vi "Update DropdownMenu.vi"(10 "VacuumLines Obj":refnum<class "VacuumLines.lvclass">, 11 "Ref of Array":refnum<vi>) -> ()   [LabVIEW 2016, in "Hardware.lvlib" / "VacuumLine.lvlib" / "VacuumLines Configuration.lvclass"]
uses:
  <userlib>/Common Components/Hardware/Abstract System/VacuumLine/VacuumLines Configuration/VacuumLines Configuration.lvclass
  <userlib>/Common Components/Hardware/Abstract System/VacuumLine/VacuumLines/VacuumLines.lvclass
  <userlib>/Common Components/Hardware/Abstract System/VacuumLine/VacuumLines/VacuumLines.lvclass/VacuumLines.ctl
  <userlib>/Common Components/Hardware/Abstract Hardware/Hardware.lvclass/Hardware.ctl
  <userlib>/Common Components/Hardware/Abstract System/VacuumLine/VacuumLine/VacuumLine.lvclass/VacuumLine.ctl
  <userlib>/Common Components/Hardware/GaugeController/GaugeController/GaugeController.lvclass
  C:/Program Files (x86)/National Instruments/LabVIEW 2016/user.lib/Common Components/Hardware/Abstract Hardware/Hardware.lvclass
  <userlib>/Common Components/Hardware/Abstract System/VacuumLine/VacuumLine/VacuumLine.lvclass
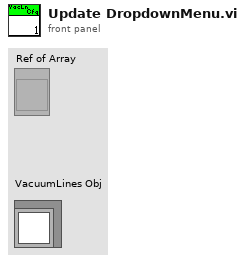
[diagram p1: front panel]
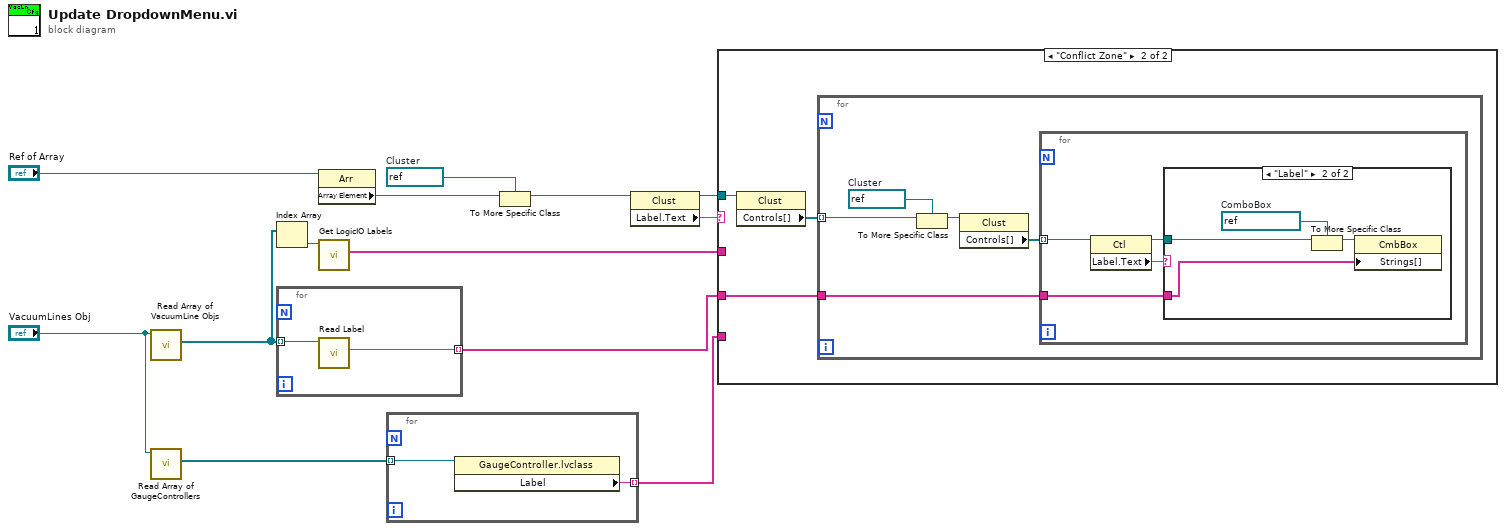
[diagram p0: block diagram]
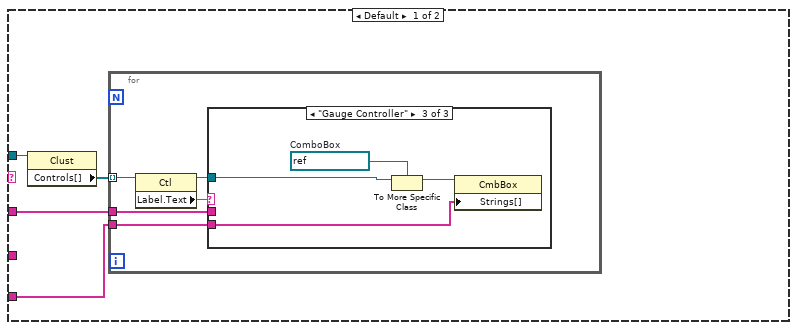
[diagram p2: hidden frame]
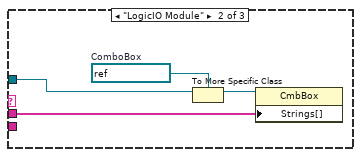
[diagram p4: hidden frame]
diagram:
  w12 = refnum<vi> refnum  # Cluster
  n1 = call <userlib>:"Read Array of VacuumLine Objs.vi"("VacuumLines in"="VacuumLines Obj") -> ("Array of VacuumLine Objs"=w4:refnum<class "VacuumLine.lvclass">[])  [unwired: 9 in, 1 out]
  n2 = call <userlib>:"Read Array of GaugeControllers.vi"("VacuumLines in"="VacuumLines Obj") -> ("Array of GaugeControllers"=w7:refnum<class "GaugeController.lvclass">[])  [unwired: 9 in, 1 out]
  n3 = Index Array(array=w4) -> (element=w8:refnum<class "VacuumLine.lvclass">)  [unwired: 1 in]
  n4 = for {
    tunnel: w4 -> [w15] mode=indexing
    tunnel: [w14] -> w3 mode=indexing
    n5 = call <userlib>:"Read Label.vi"("VacuumLine in"=w15) -> ("Label"=w14:string)  [unwired: 8 in, 2 out]
  }
  n6 = property class="Arr"(reference="Ref of Array") -> ("Array Element"=w11:refnum<vi>)  [unwired: 1 in, 2 out]
  n7 = call <userlib>:"Get LogicIO Labels.vi"("VacuumLine in"=w8) -> ("LogicIO Labels"=w13:string[])  [unwired: 8 in, 2 out]
  n8 = for {
    tunnel: w7 -> [w17] mode=indexing
    tunnel: [w16] -> w6 mode=indexing
    n9 = property class="GaugeController.lvclass"(reference=w17) -> ("Label"=w16:string)  [unwired: 1 in, 2 out]
  }
  n10 = To More Specific Class(target class=w12, reference=w11) -> (specific class reference=w10:refnum<vi>)  [unwired: 1 in, 1 out]
  n11 = property class="Clust"(reference=w10) -> (reference out=w2:refnum<vi>, "Label.Text"=w1:string)  [unwired: 1 in, 1 out]
  n12 = case shown="\"Conflict Zone\"" w1 {
    tunnel: w13 -> [w21 _]
    tunnel: w6 -> [w19 _]
    tunnel: w3 -> [_ w35]
    tunnel: w2 -> [w18 w36]
    frame Default {
      n13 = property class="Clust"(reference=w18) -> ("Controls[]"=w20:refnum<vi>[])  [unwired: 1 in, 2 out]
      n14 = for {
        tunnel: w20 -> [w26] mode=indexing
        tunnel: w21 -> [w23]
        tunnel: w19 -> [w22]
        n15 = property class="Ctl"(reference=w26) -> (reference out=w24:refnum<vi>, "Label.Text"=w25:string)  [unwired: 1 in, 1 out]
        n16 = case shown="\"Gauge Controller\"" w25 {
          tunnel: w24 -> [_ w28 w32]
          tunnel: w23 -> [_ w27 _]
          tunnel: w22 -> [_ _ w31]
          frame Default {
          }
          frame "LogicIO Module" {
            w30 = refnum<vi> refnum  # ComboBox
            n17 = To More Specific Class(target class=w30, reference=w28) -> (specific class reference=w29:refnum<vi>)  [unwired: 1 in, 1 out]
            n18 = property class="CmbBox"(reference=w29, "Strings[]"=w27) -> ()  [unwired: 1 in, 2 out]
          }
          frame "Gauge Controller" {
            w34 = refnum<vi> refnum  # ComboBox
            n19 = To More Specific Class(target class=w34, reference=w32) -> (specific class reference=w33:refnum<vi>)  [unwired: 1 in, 1 out]
            n20 = property class="CmbBox"(reference=w33, "Strings[]"=w31) -> ()  [unwired: 1 in, 2 out]
          }
        }
      }
    }
    frame "Conflict Zone" {
      n21 = property class="Clust"(reference=w36) -> ("Controls[]"=w37:refnum<vi>[])  [unwired: 1 in, 2 out]
      n22 = for {
        tunnel: w37 -> [w39] mode=indexing
        tunnel: w35 -> [w42]
        w41 = refnum<vi> refnum  # Cluster
        n23 = To More Specific Class(target class=w41, reference=w39) -> (specific class reference=w40:refnum<vi>)  [unwired: 1 in, 1 out]
        n24 = property class="Clust"(reference=w40) -> ("Controls[]"=w38:refnum<vi>[])  [unwired: 1 in, 2 out]
        n25 = for {
          tunnel: w42 -> [w44]
          tunnel: w38 -> [w43] mode=indexing
          n26 = property class="Ctl"(reference=w43) -> (reference out=w45:refnum<vi>, "Label.Text"=w46:string)  [unwired: 1 in, 1 out]
          n27 = case shown="\"Label\"" w46 {
            tunnel: w45 -> [_ w48]
            tunnel: w44 -> [_ w47]
            frame Default {
            }
            frame "Label" {
              w50 = refnum<vi> refnum  # ComboBox
              n28 = To More Specific Class(target class=w50, reference=w48) -> (specific class reference=w49:refnum<vi>)  [unwired: 1 in, 1 out]
              n29 = property class="CmbBox"(reference=w49, "Strings[]"=w47) -> ()  [unwired: 1 in, 2 out]
            }
          }
        }
      }
    }
  }
